vi "Stop Config.vi"(2 "OldVal":i32, 3 "Array":T1[](array[typedef]) {"Private"."Offset" format="%^_3e"; "Private"."Scale Factors" format="%^_3e"}) -> (1 "Array Out":T1[](array[typedef]) {"Private"."Offset" format="%^_3e"; "Private"."Scale Factors" format="%^_3e"})   [LabVIEW 2025]
doc: "Author: Scott Hannahs <sth@magnet.fsu.edu>\n\nThis software is licensed for use under the “MIT License\"\nCopyright (c) 2025 Scott Hannahs, sth@sth@magnet.sthnet.net\n\nPermission is hereby granted, free of charge, to any person obtaining a copy of this software and associated documentation files (the \"Software\"), to deal in the Software without restriction, including without limitation the rights to use, copy, modify, merge, publish, distribute, sublicense, and/or sell copies of the Software, and to permit persons to whom the Software is furnished to do so, subject to the following conditions: The above copyright notice and this permission notice shall be included in all copies or substantial portions of the Software.\n\nTHE SOFTWARE IS PROVIDED \"AS IS\", WITHOUT WARRANTY OF ANY KIND, EXPRESS OR IMPLIED, INCLUDING BUT NOT LIMITED TO THE WARRANTIES OF MERCHANTABILITY, FITNESS FOR A PARTICULAR PURPOSE AND NONINFRINGEMENT. IN NO EVENT SHALL THE AUTHORS OR COPYRIGHT HOLDERS BE LIABLE FOR ANY CLAIM, DAMAGES OR OTHER LIABILITY, WHETHER IN AN ACTION OF CONTRACT, TORT OR OTHERWISE, ARISING FROM, OUT OF OR IN CONNECTION WITH THE SOFTWARE OR THE USE OR OTHER DEALINGS IN THE SOFTWARE."
uses:
  New NML Data Acq/Sub Controls/Instrument Properties.ctl
  New NML Data Acq/Sub Controls/Public.ctl
  New NML Data Acq/Sub Controls/Private.ctl
  New NML Data Acq/Sub Controls/Instrument Ref.ctl
  New NML Data Acq/Sub Controls/SystemCheckBox-resize.ctl
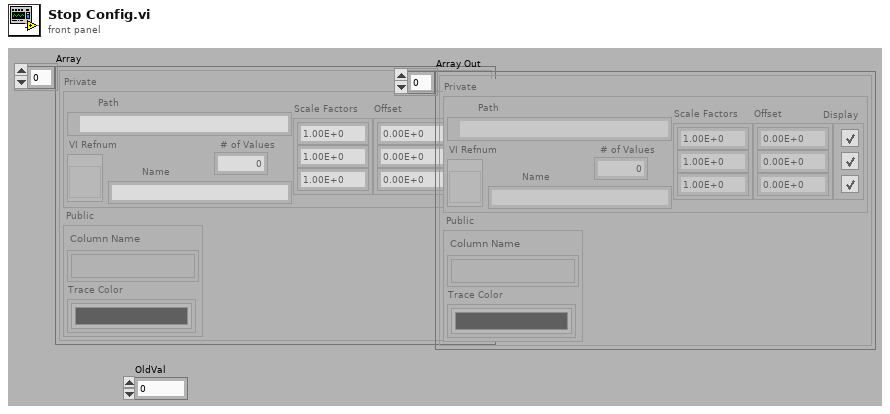
[diagram p1: front panel]
types:
  T1 = typedef "Instrument Properties.ctl" = cluster{"Public":T2, "Private":T3}
  T2 = typedef "Public.ctl" = cluster{"Column Name":string[], "Trace Color":u32[]}
  T3 = typedef "Private.ctl" = cluster{"Path":path, "VI Refnum":T4, "Name":string, "# of Values":i32, "Scale Factors":dbl[], "Display":T5[], "Offset":dbl[]}
  T4 = typedef "Instrument Ref.ctl" = refnum<vi>
  T5 = typedef "SystemCheckBox-resize.ctl" = bool
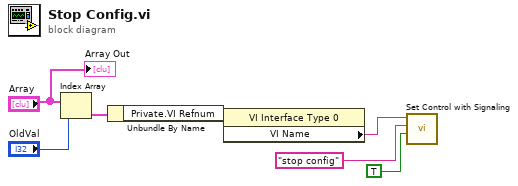
[diagram p0: block diagram]
diagram:
  n1 = Index Array(array="Array", index="OldVal") -> (element=w6:T1)
  n2 = Unbundle By Name(w6) -> ("Private.VI Refnum"=w4:T4)
  n3 = property class="VI Interface Type 0"(reference=w4) -> ("VI Name"=w1:string)  [unwired: 1 in, 2 out]
  n4 = call "Set Control with Signaling.vi"("Value"=TRUE, "Control Name"="stop config" ("y"), "VI Name"=w1) -> ()  [unwired: 8 in, 1 out]
  "Array Out" <- "Array"
